vi "Limits Configurator.vi"() -> ()   [LabVIEW 2024]
doc: "Use this configurator to build a limits file based on specific sequence file. Uses the sequence file name to generate the limits file neame because they are paired."
uses:
  <vilib>/addons/_JKI Toolkits/State Machine/_JKI_lib_State_Machine.llb/Select State(s)_err__jki_lib_state_machine.vi
  <vilib>/addons/_JKI Toolkits/State Machine/_JKI_lib_State_Machine.llb/Periodic Trigger__ogtk__JKI-SM__jki_lib_state_machine.vi
  <userlib>/_OpenG.lib/file/file.llb/Convert File Extension (String)__ogtk.vi
  <userlib>/_OpenG.lib/file/file.llb/File Exists - Scalar__ogtk.vi
  <vilib>/Utility/file.llb/Write Delimited Spreadsheet (string).vi
  <vilib>/Utility/file.llb/Read Delimited Spreadsheet (string).vi
  <userlib>/_OpenG.lib/appcontrol/appcontrol.llb/openg_application_control.lvlib
  <userlib>/_OpenG.lib/file/file.llb/openg_file.lvlib
panel:
  in  "Remove Button":bool
  in  "Sequence File Path":path
  in  "Close Button":bool
  in  "Limits Table":i32(listbox)
  in  "Add Button":bool
  in  "Test Cases":u16(ring) items=["Connect Test", "PSU Test", "LED Test", "Firmware Test", "Shutdown"]
  # "LIMITS CONFIGURATOR"
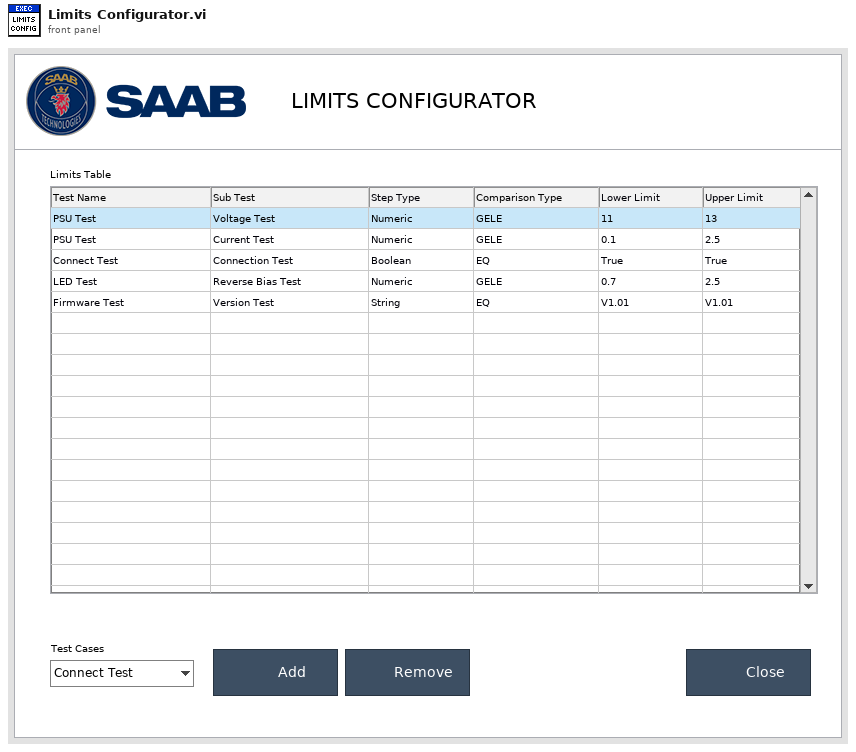
[diagram p1: front panel]
types:
  T1 = enum32{"Invalid", "Standard", "Closed", "Hidden", "Minimized", "Maximized"}
  T2 = enum32{"invalid app kind", "Development System", "Run Time System", "Student Edition", "Embedded LabVIEW", "Evaluation", "Custom"}
  T3 = enum8{"Enabled", "Disabled", "Disabled and Grayed Out"}
  T4 = cluster{"Core":cluster{"Current VI Reference":refnum<vi>, "Close Panel on Exit?":bool}, "Sequence File Path":path, "Limit Data Array":string[][], "Limits File Path":path}
  T5 = cluster{"Current VI Reference":refnum<vi>, "Close Panel on Exit?":bool}
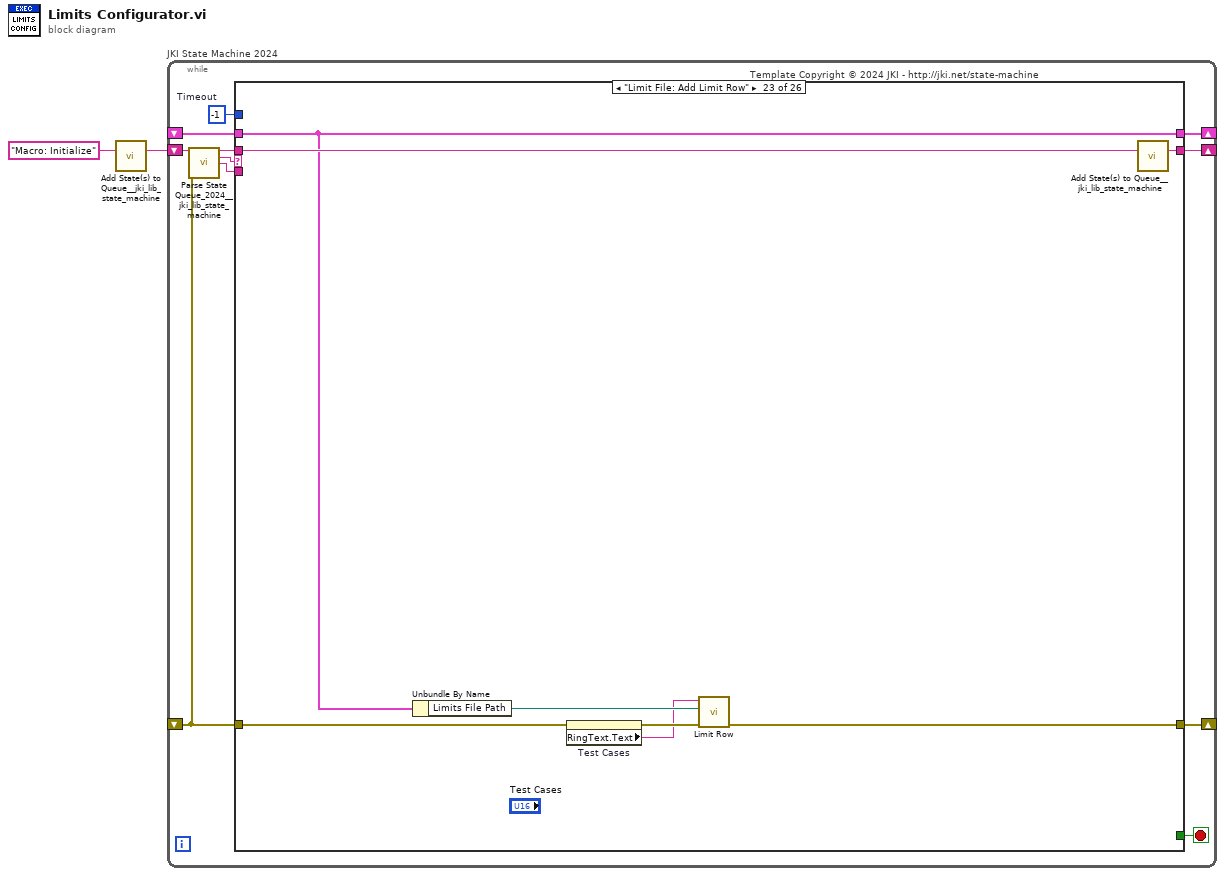
[diagram p0: block diagram]
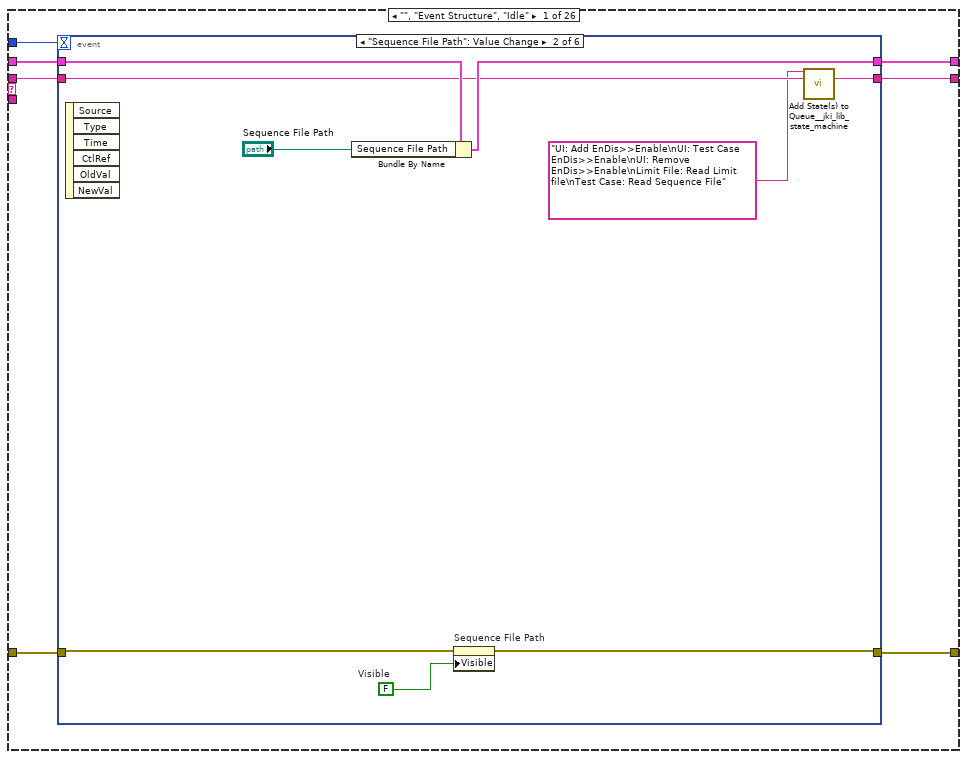
[diagram p2: hidden frame]
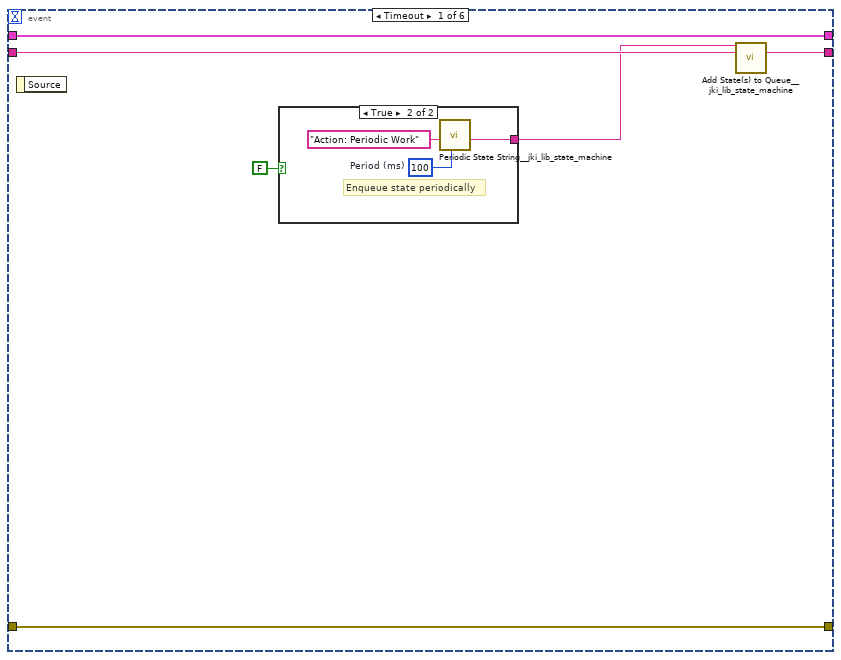
[diagram p3: hidden frame]
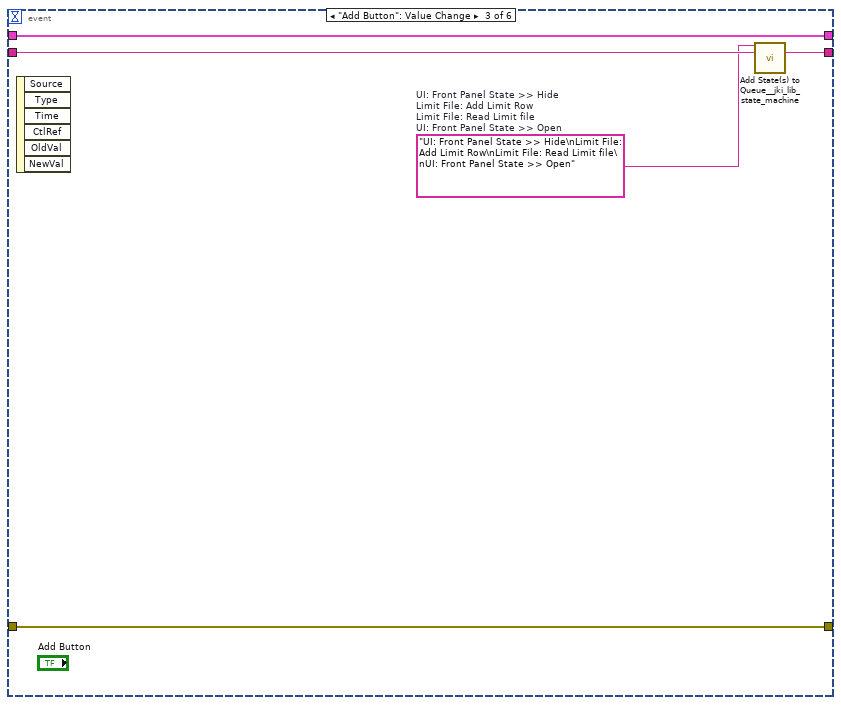
[diagram p5: hidden frame]
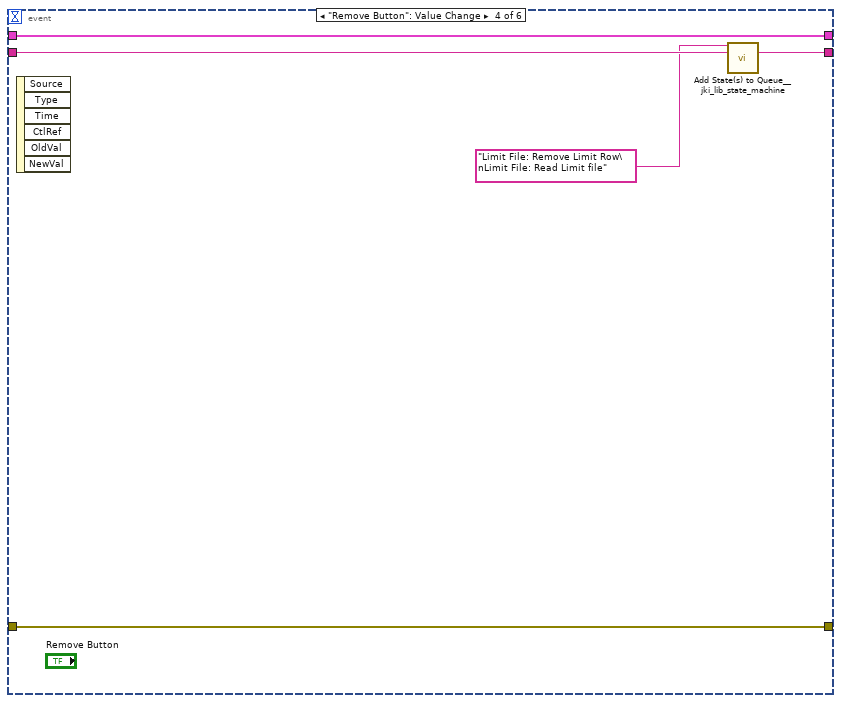
[diagram p6: hidden frame]
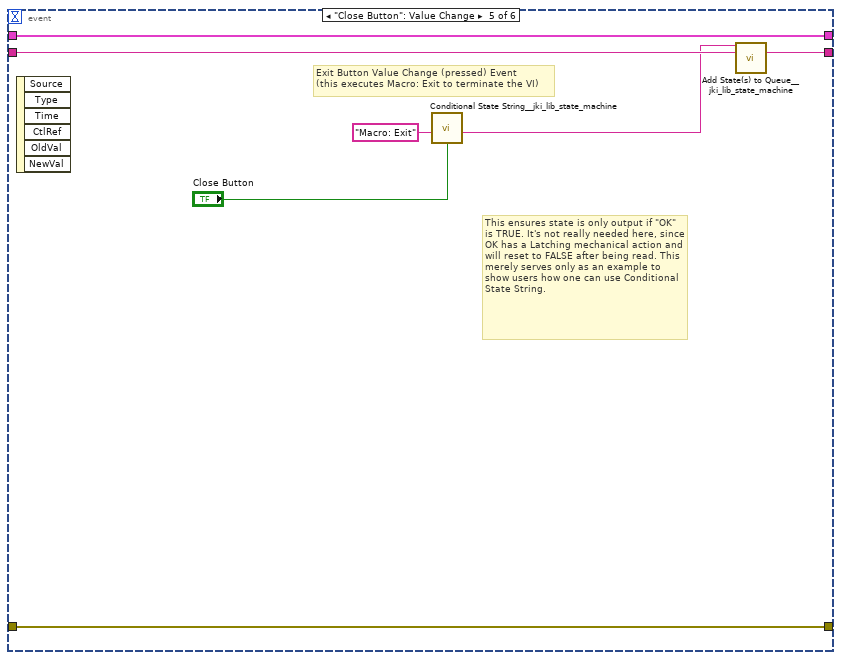
[diagram p7: hidden frame]
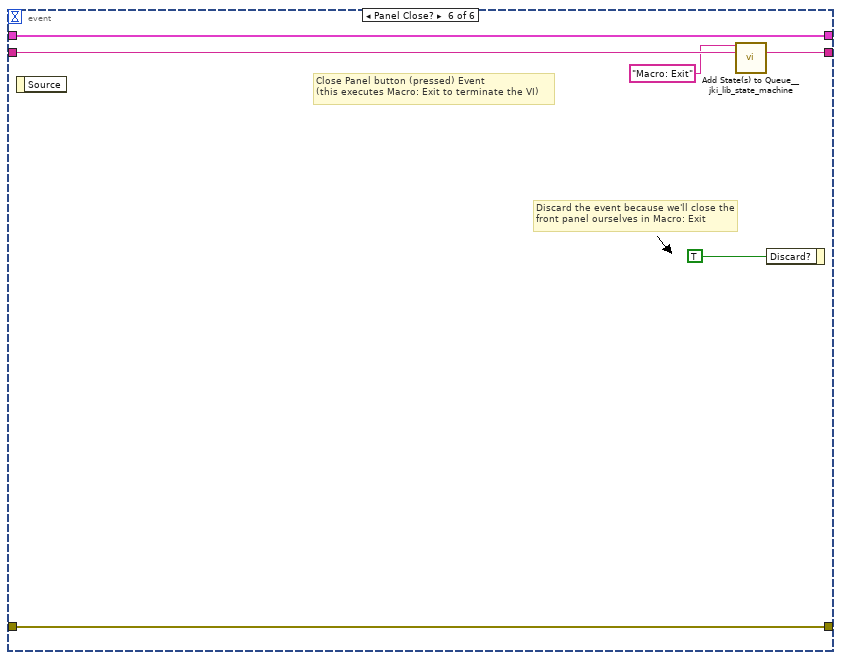
[diagram p8: hidden frame]
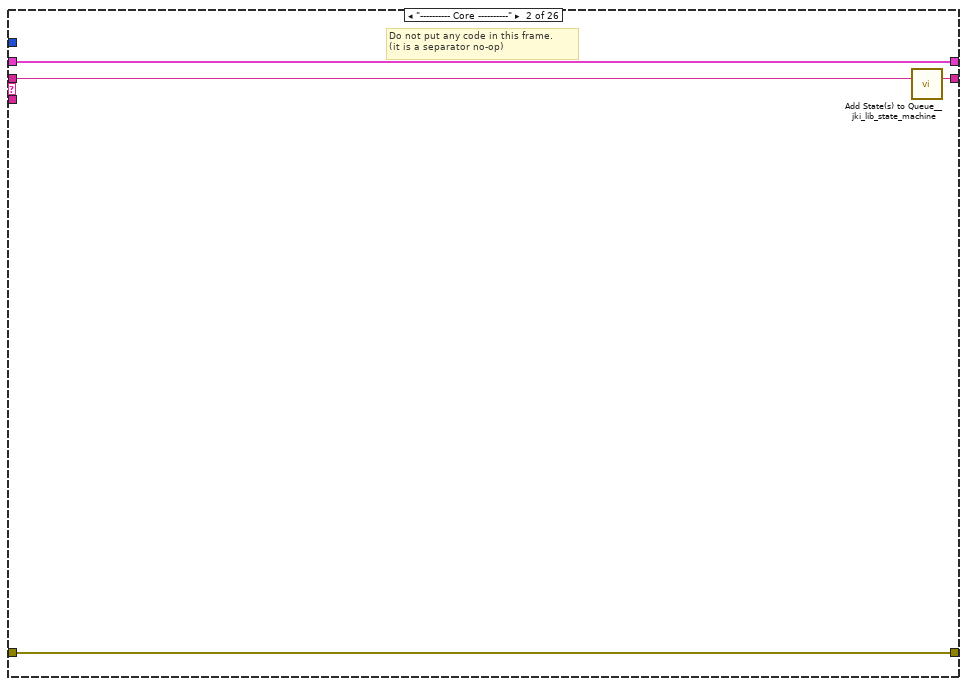
[diagram p9: hidden frame]
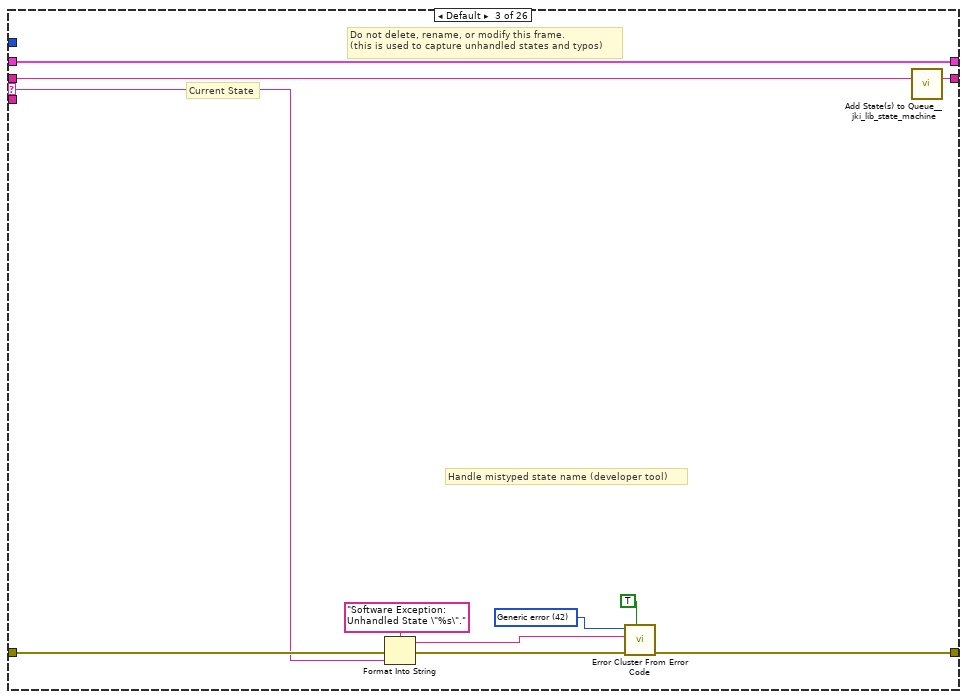
[diagram p10: hidden frame]
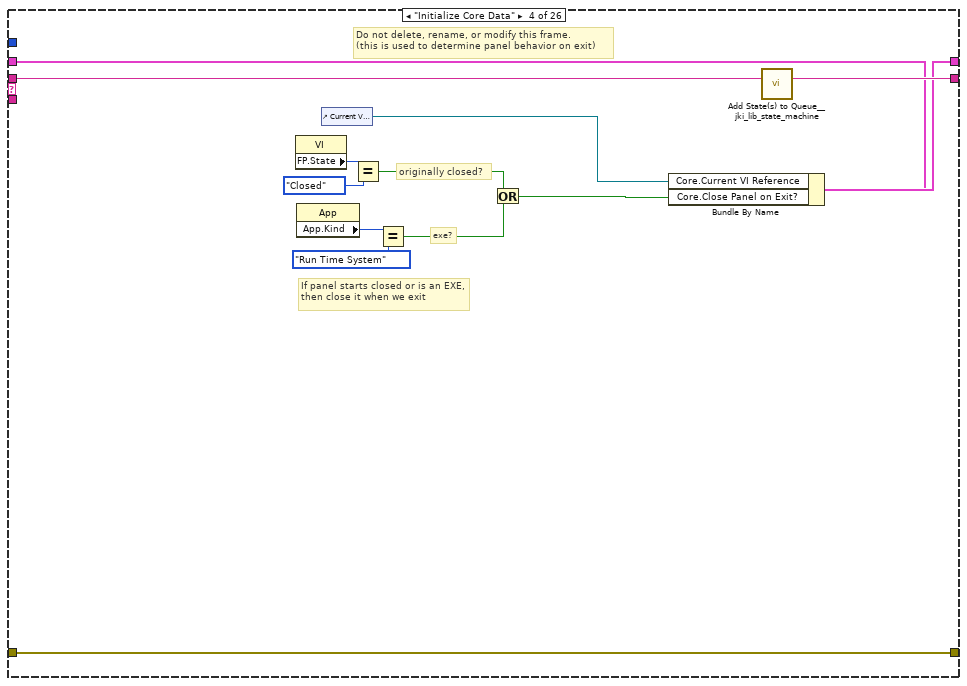
[diagram p11: hidden frame]
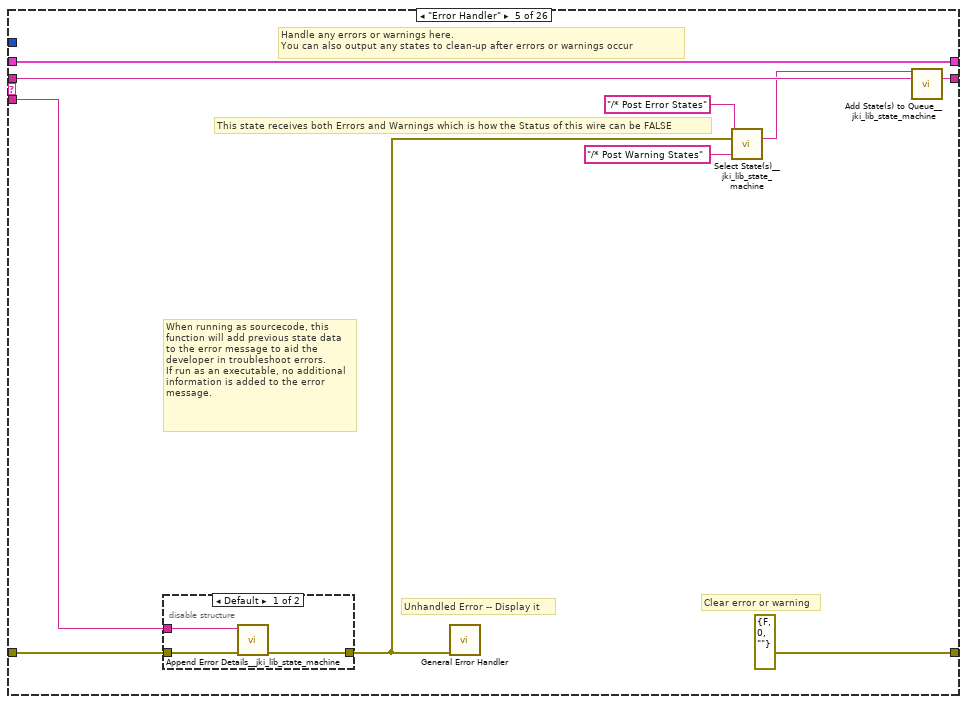
[diagram p12: hidden frame]
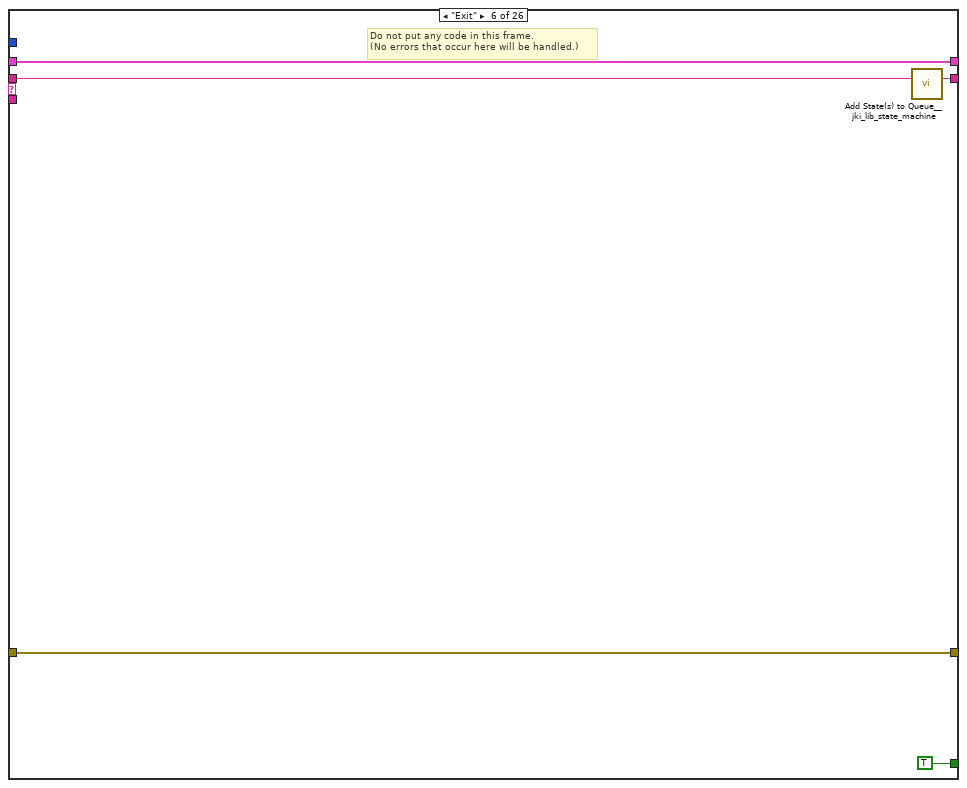
[diagram p14: hidden frame]
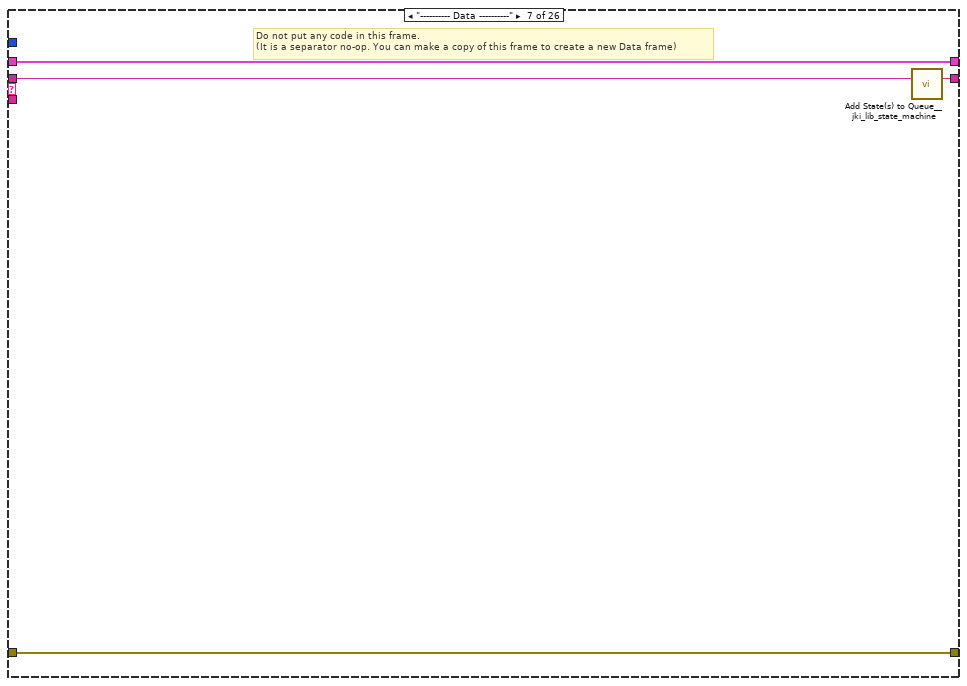
[diagram p15: hidden frame]
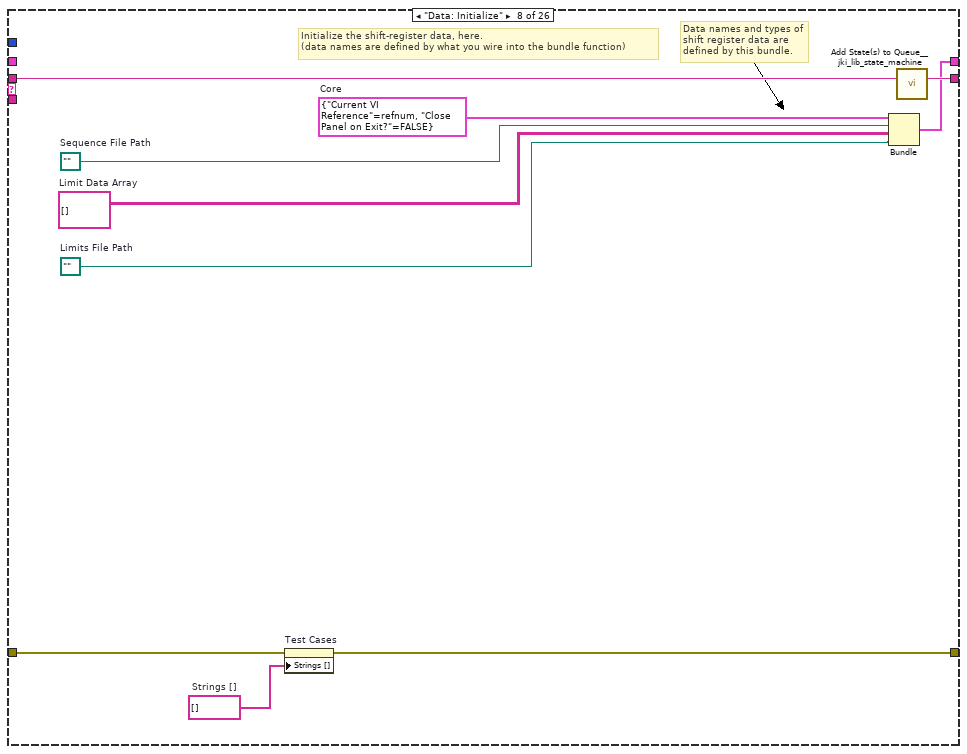
[diagram p16: hidden frame]
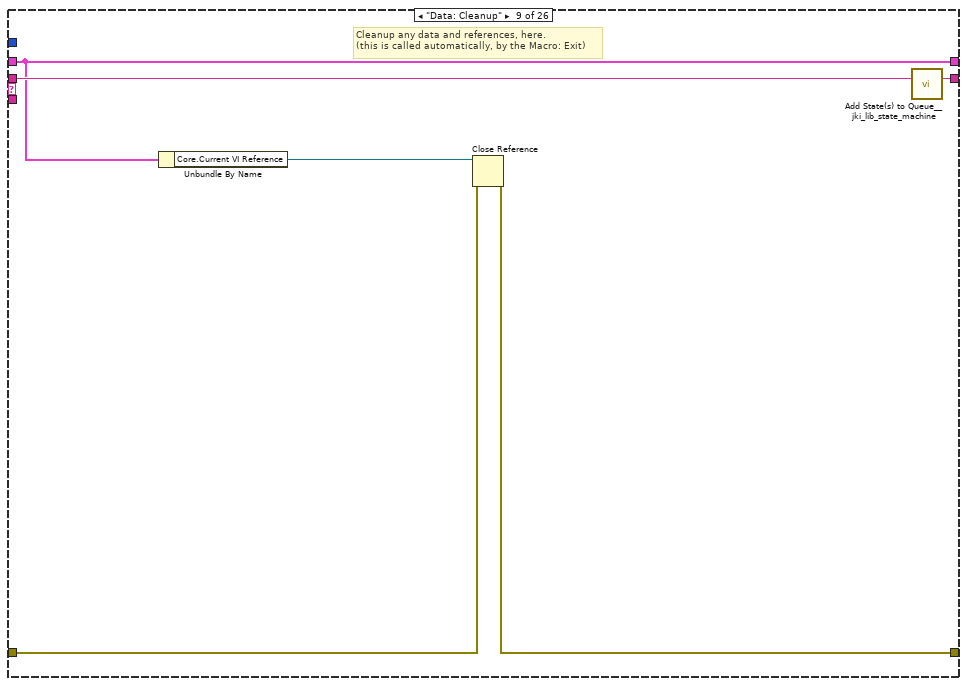
[diagram p17: hidden frame]
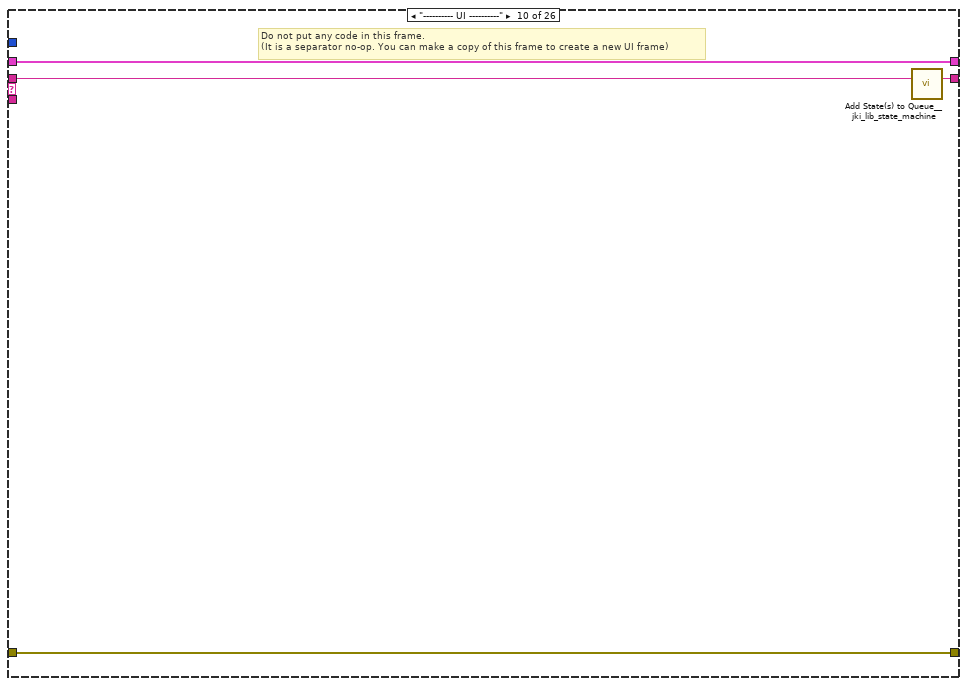
[diagram p18: hidden frame]
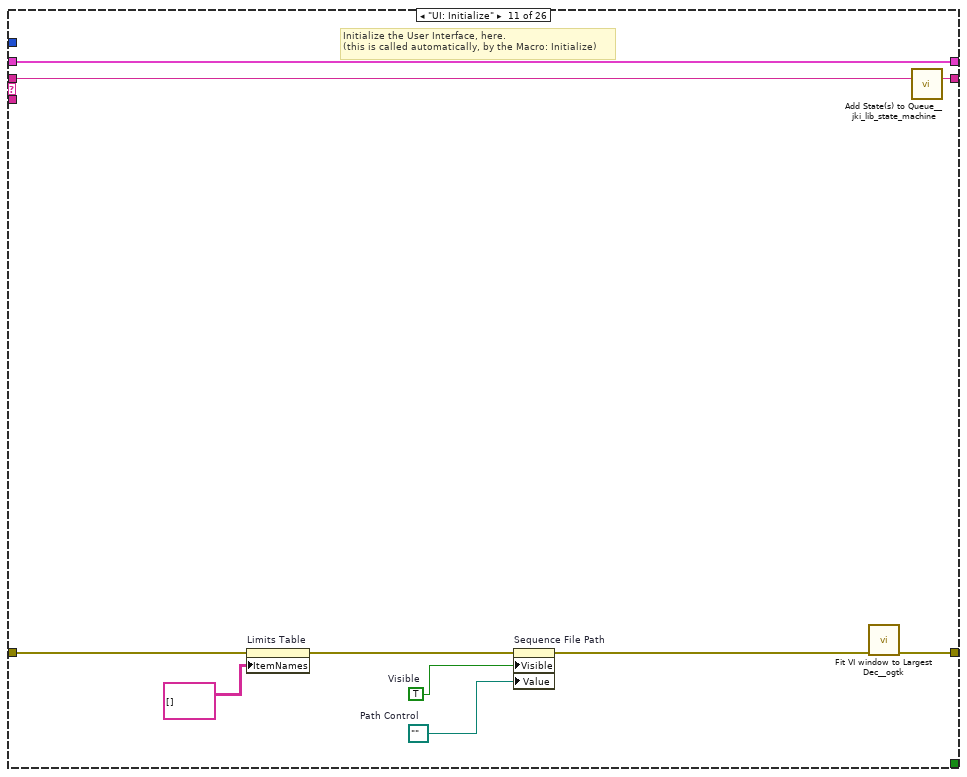
[diagram p19: hidden frame]
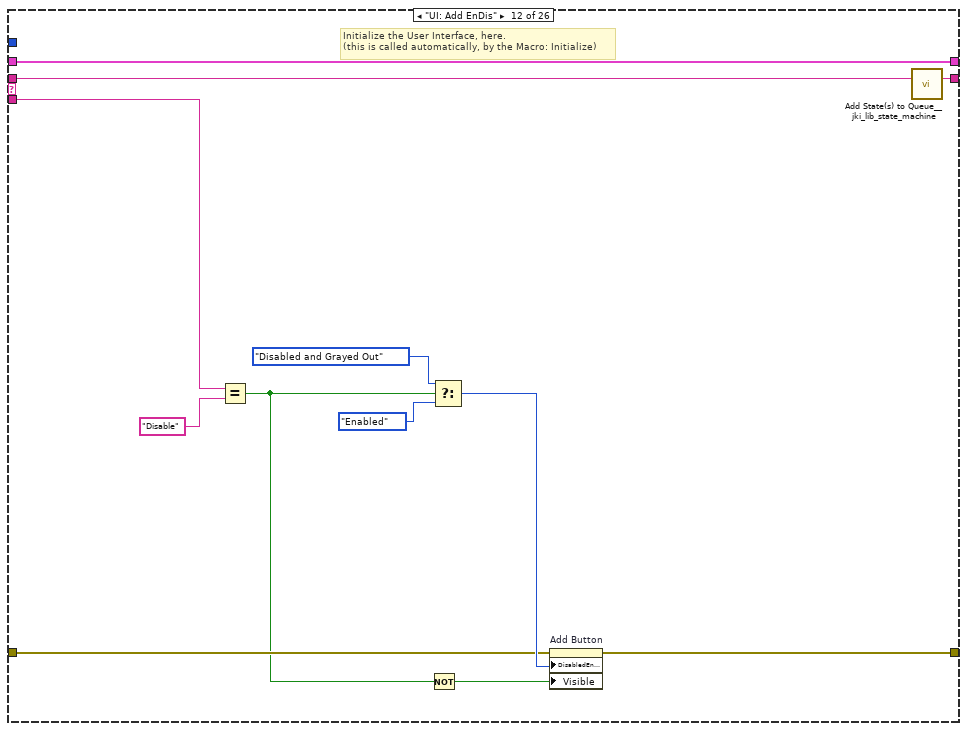
[diagram p20: hidden frame]
diagram:
  n1 = call <vilib>:"Add State(s) to Queue__jki_lib_state_machine.vi"("State(s) in (\"\")"="Macro: Initialize") -> ("States Out"=w2:string)  [unwired: 14 in]
  n2 = while "JKI State Machine 2024" {
    shift-right: [w6] -> _
    shift-left: _ -> [w5]
    shift-right: [w9] -> _
    shift-left: _ -> [w3]
    shift-right: [w8] -> _
    shift-left: w2 -> [w10]
    stop <- w7 stop-if-true
    w4 = -1  # Timeout
    # "Template Copyright © 2024 JKI - http://jki.net/state-machine"
    n3 = call <vilib>:"Parse State Queue_2024__jki_lib_state_machine.vi"("State Queue"=w10, "Error In (no error)"=w3) -> ("Remaining States"=w12:string, "Current State"=w13:string, "Arguments"=w11:string)  [unwired: 11 in]
    n4 = case shown="\"Limit File: Add Limit Row\"" w13 {
      selector: w13 -> [_ _ w66 _ _ _ _ _ _ _ _ _ _ _ _ _ _ _ _ _ _ _ _ _ _ _]
      tunnel: w12 -> [w20 w65 w70 w89 w99 w108 w112 w122 w128 w132 w142 w154 w166 w178 w182 w188 w199 w268 w273 w282 w286 w306 w328 w335 w351 w360]
      tunnel: w11 -> [_ _ _ _ w94 _ _ _ _ _ _ w146 w158 w170 _ w183 w193 _ _ _ _ _ _ _ _ _]
      tunnel: w5 -> [w18 w62 w68 w82 w96 w106 w109 _ w123 w129 w140 w152 w164 w176 w180 w186 w195 w265 w270 w280 w283 w289 w325 w333 w348 w353]
      tunnel: [w17 w63 w72 w86 errorcluster {"status"=FALSE, "code"=0, "source"=""} ("error out") w105 w110 w115 w124 w130 w139 w147 w159 w171 w179 w184 w196 w266 w271 w277 w284 w302 w326 w331 w349 w358] -> w9
      tunnel: w3 -> [w14 w63 w71 w86 w95 w105 w110 w114 w125 w130 w138 w145 w157 w169 w179 w185 w197 w266 w271 w277 w284 w304 w322 w332 w349 w357]
      tunnel: [w19 w64 w69 w88 w98 w107 w111 w121 w127 w131 w141 w153 w165 w177 w181 w187 w198 w267 w272 w281 w285 w305 w327 w334 w350 w359] -> w8
      tunnel: [_ _ _ _ _ TRUE _ _ _ _ _ _ _ _ _ _ _ _ _ _ _ _ _ _ _ _] -> w7
      tunnel: [w16 w62 w68 w87 w96 w106 w109 w120 w123 w129 w140 w152 w164 w176 w180 w186 w195 w265 w270 w280 w283 w288 w325 w333 w348 w353] -> w6
      tunnel: w4 -> [w15 _ _ _ _ _ _ _ _ _ _ _ _ _ _ _ _ _ _ _ _ _ _ _ _ _]
      frame "", "Event Structure", "Idle" {
        n5 = event shown="[1] \"Sequence File Path\": Value Change" {
          selector: _ -> [_ _ _ _ _ _]
          dyn-events: _ -> [_ _ _ _ _ _]
          timeout: w15 -> [_ _ _ _ _ _]
          tunnel: w20 -> [w26 w34 w41 w45 w55 w61]
          tunnel: [w25 w35 w42 w46 w54 w60] -> w19
          tunnel: w18 -> [w23 w38 w39 w47 w52 w58]
          tunnel: [w24 w32 w43 w48 w53 w59] -> w17
          tunnel: w14 -> [w24 w31 w43 w48 w53 w59]
          tunnel: [w23 w37 w39 w47 w52 w58] -> w16
          event Timeout {
            n6 = event-data() -> ()  [unwired: 1 in, 1 out]
            n7 = case shown="True" FALSE {
              tunnel: [_ w29] -> w22
              frame False {
              }
              frame True {
                w27 = u32 100  # Period (ms)
                # "Enqueue state periodically"
                n8 = call <vilib>:"Periodic State String__jki_lib_state_machine.vi"("Period (ms)"=w27, "State"="Action: Periodic Work") -> ("State Out"=w29:string)  [unwired: 9 in]
              }
            }
            n9 = call <vilib>:"Add State(s) to Queue__jki_lib_state_machine.vi"("State(s) in Front (\"\")"=w22, "State(s) in (\"\")"=w26) -> ("States Out"=w25:string)  [unwired: 13 in]
          }
          event "Sequence File Path": Value Change {
            w30 = FALSE  # Visible
            n10 = event-data() -> ()  [unwired: 1 in, 6 out]
            n11 = Bundle By Name(cluster=w38, "Sequence File Path"="Sequence File Path") -> (w37:T4)
            n12 = property on="Sequence File Path" class="Path"(error in=w31, "Visible"=w30) -> (error out=w32:errorcluster)  [unwired: 1 in, 1 out]
            n13 = call <vilib>:"Add State(s) to Queue__jki_lib_state_machine.vi"("State(s) in Front (\"\")"="UI: Add EnDis>>Enable\nUI: Test Case EnDis>>Enable\nUI: Remove EnDis>>Enable\nLimit File: Read Limit file\nTest Case: Read Sequence File", "State(s) in (\"\")"=w34) -> ("States Out"=w35:string)  [unwired: 13 in]
          }
          event "Add Button": Value Change {
            w40 = "UI: Front Panel State >> Hide\nLimit File: Add Limit Row\nLimit File: Read Limit file\nUI: Front Panel State >> Open"  # UI: Front Panel State >> Hide Limit File: Add Limit Row Limit File: Read Limit file UI: Front Panel State >> Open
            n14 = event-data() -> ()  [unwired: 1 in, 6 out]
            n15 = call <vilib>:"Add State(s) to Queue__jki_lib_state_machine.vi"("State(s) in Front (\"\")"=w40, "State(s) in (\"\")"=w41) -> ("States Out"=w42:string)  [unwired: 13 in]
          }
          event "Remove Button": Value Change {
            n16 = event-data() -> ()  [unwired: 1 in, 6 out]
            n17 = call <vilib>:"Add State(s) to Queue__jki_lib_state_machine.vi"("State(s) in Front (\"\")"="Limit File: Remove Limit Row\nLimit File: Read Limit file", "State(s) in (\"\")"=w45) -> ("States Out"=w46:string)  [unwired: 13 in]
          }
          event "Close Button": Value Change {
            # "This ensures state is only output if \"OK\" is TRUE. It's not really needed here, since OK has a Latching mechanical action and will reset to FALSE after being read. This merely serves only as an example to show users how one can use Conditional State String."
            # "Exit Button Value Change (pressed) Event\n(this executes Macro: Exit to terminate the VI)"
            n18 = event-data() -> ()  [unwired: 1 in, 6 out]
            n19 = call <vilib>:"Conditional State String__jki_lib_state_machine.vi"("Do State(s)?"="Close Button", "State"="Macro: Exit") -> ("State Out"=w50:string)  [unwired: 7 in]
            n20 = call <vilib>:"Add State(s) to Queue__jki_lib_state_machine.vi"("State(s) in Front (\"\")"=w50, "State(s) in (\"\")"=w55) -> ("States Out"=w54:string)  [unwired: 13 in]
          }
          event Panel Close? {
            # "Discard the event because we'll close the front panel ourselves in Macro: Exit"
            # "Close Panel button (pressed) Event\n(this executes Macro: Exit to terminate the VI)"
            n21 = event-data() -> ()  [unwired: 1 in, 1 out]
            n22 = call <vilib>:"Add State(s) to Queue__jki_lib_state_machine.vi"("State(s) in Front (\"\")"="Macro: Exit", "State(s) in (\"\")"=w61) -> ("States Out"=w60:string)  [unwired: 13 in]
            n23 = event-data("Discard?"=TRUE) -> ()  [unwired: 1 in, 1 out]
          }
        }
      }
      frame "---------- Core ----------" {
        # "Do not put any code in this frame.\n(it is a separator no-op)"
        n24 = call <vilib>:"Add State(s) to Queue__jki_lib_state_machine.vi"("State(s) in (\"\")"=w65) -> ("States Out"=w64:string)  [unwired: 14 in]
      }
      frame Default {
        w75 = 42 items=["No error", "Argument error", "Memory is full", "Out of zone", "End of file", "File already open", "Generic file I/O error", "File not found", "File permission error", "Disk is full", "Duplicate path", "Too many files open", "System feature not enabled", "Resource file not found", "Cannot add resource", "Resource not found", "Image not found", "Image memory error", "Pen does not exist", "Config type invalid", "Config token not found", "Config parse error", "Config memory error", "Bad external code format", "Bad external code offset", "External code not present", "Null window", "Destroy window error", "Null menu", "Print aborted", "Bad print record", "Print driver error", "Windows error during printing", "Memory error during printing", "Print dialog error", "Generic print error", "Invalid device refnum", "Device not found", "Device parameter error", "Device unit error", "Cannot open device", "Device call aborted", "Generic error", "Cancelled by user", "Object ID too low", "Object ID too high", "Object not in heap", "Unknown heap", "Unknown object (invalid DefProc)", "Unknown object (DefProc not in table)", "Message out of range", "Invalid (null) method", "Unknown message", "Manager call not supported", "Bad address", "Network operation in progress", "Network operation timed out", "Connection is busy", "Network attribute not supported", "Network error", "Address in use", "System out of memory", "Connection aborted", "Connection refused", "Not connected", "Already connected", "Connection closed", "Initialization error (interapplication manager)", "Bad occurrence", "Wait on unbound occurrence handler", "Occurrence queue overflow", "Datalog type conflict", "Unused", "Unrecognized type (interapplication manager)", "Memory corrupt", "Failed to make temporary DLL", "Old CIN version", "Drag socket not found", "Failed to load drop-object", "Failed to register OLE object", "Failed to release OLE object", "Format specifier type mismatch", "Unknown format specifier", "Too few format specifiers", "Too many format specifiers", "Scan failed", "Newer CIN version", "Error converting to variant", "Runtime menu error", "Password tampered", "Variant attribute not found", "Incompatible variant data type", "Event data is not available", "Event Store is not present", "Occurrence is not found", "Event Queue is not created", "Event info is not available", "Refnum passed is NULL", "Error retrieving Class GUID", "Error retrieving CoClass GUID", "Error retrieving TypeLib GUID.", "Bad built application magic bytes.", "Specific driver is different from the specific driver associated with the Logical Name.", "There is no session opened to the class driver.", "Max Error", "MAX - Error with config objects", "MAX - Error loading configuration", "MAX - Group not supported"]
        # "Current State"
        # "Do not delete, rename, or modify this frame.\n(this is used to capture unhandled states and typos)"
        # "Handle mistyped state name (developer tool)"
        n25 = Format Into String(format string="Software Exception: Unhandled State \"%s\"." ("message"), error in=w71, w66) -> (resulting string=w74:string, error out=w73:errorcluster)  [unwired: 1 in]
        n26 = call <vilib>:"Error Cluster From Error Code.vi"("show call chain? (False)"=TRUE, "error in (no error)"=w73, "error message (\"\")"=w74, "error code (0)"=w75) -> ("error out"=w72:errorcluster)  [unwired: 5 in]
        n27 = call <vilib>:"Add State(s) to Queue__jki_lib_state_machine.vi"("State(s) in (\"\")"=w70) -> ("States Out"=w69:string)  [unwired: 14 in]
      }
      frame "Initialize Core Data" {
        # "Do not delete, rename, or modify this frame.\n(this is used to determine panel behavior on exit)"
        # "originally closed?"
        # "exe?"
        # "If panel starts closed or is an EXE, then close it when we exit"
        n28 = property class="VI"() -> ("FP.State"=w79:T1)  [unwired: 2 in, 2 out]
        n29 = property class="App"() -> ("App.Kind"=w85:T2)  [unwired: 2 in, 2 out]
        n30 = control-ref of="Current VI Reference"() -> (w80:refnum<vi>)
        n31 = Equal?(x=w79, y=T1."Closed" ("Front Panel Window:State")) -> (x = y?=w77:bool)
        n32 = Equal?(x=w85, y=T2."Run Time System" ("Application:Kind")) -> (x = y?=w83:bool)
        n33 = Or(x=w77, y=w83) -> (x .or. y?=w81:bool)
        n34 = Bundle By Name(cluster=w82, "Core.Current VI Reference"=w80, "Core.Close Panel on Exit?"=w81) -> (w87:T4)
        n35 = call <vilib>:"Add State(s) to Queue__jki_lib_state_machine.vi"("State(s) in (\"\")"=w89) -> ("States Out"=w88:string)  [unwired: 14 in]
      }
      frame "Error Handler" {
        # "When running as sourcecode, this function will add previous state data to the error message to aid the developer in troubleshoot errors.\nIf run as an executable, no additional information is added to the error message."
        # "This state receives both Errors and Warnings which is how the Status of this wire can be FALSE"
        # "Unhandled Error -- Display it"
        # "Handle any errors or warnings here.\nYou can also output any states to clean-up after errors or warnings occur"
        # "Clear error or warning"
        n36 = disable-structure shown="Default" {
          disable-tunnel: w95 -> [w102 w103]
          disable-tunnel: w94 -> [w101 _]
          disable-tunnel: [w100 w103] -> w93
          frame condition #0 (active) {
            n37 = call <vilib>:"Append Error Details__jki_lib_state_machine.vi"("error in (no error)"=w102, "Previous State and Argument(s)"=w101) -> ("error out"=w100:errorcluster)  [unwired: 9 in]
          }
          frame condition #1 {
          }
        }
        n38 = call <vilib>:"General Error Handler.vi"("error in (no error)"=w93) -> ()  [unwired: 10 in, 5 out]
        n39 = call-poly <vilib>:"Select State(s)__jki_lib_state_machine.vi"("State(s) if True (\"\")"="/* Post Error States", "Select"=w93, "State(s) if False (\"\")"="/* Post Warning States") -> ("States Out"=w91:string)  [unwired: 12 in]
        n40 = call <vilib>:"Add State(s) to Queue__jki_lib_state_machine.vi"("State(s) in Front (\"\")"=w91, "State(s) in (\"\")"=w99) -> ("States Out"=w98:string)  [unwired: 13 in]
      }
      frame "Exit" {
        # "Do not put any code in this frame.\n(No errors that occur here will be handled.)"
        n41 = call <vilib>:"Add State(s) to Queue__jki_lib_state_machine.vi"("State(s) in (\"\")"=w108) -> ("States Out"=w107:string)  [unwired: 14 in]
      }
      frame "---------- Data ----------" {
        # "Do not put any code in this frame.\n(It is a separator no-op. You can make a copy of this frame to create a new Data frame)"
        n42 = call <vilib>:"Add State(s) to Queue__jki_lib_state_machine.vi"("State(s) in (\"\")"=w112) -> ("States Out"=w111:string)  [unwired: 14 in]
      }
      frame "Data: Initialize" {
        w113 = string[] []  # Strings []
        w116 = path ""  # Limits File Path
        w117 = string[][] []  # Limit Data Array
        w118 = path ""  # Sequence File Path
        w119 = T5 {"Current VI Reference"=refnum, "Close Panel on Exit?"=FALSE}  # Core
        # "Data names and types of shift register data are defined by this bundle."
        # "Initialize the shift-register data, here.\n(data names are defined by what you wire into the bundle function)"
        n43 = property on="Test Cases" class="Ring (strict)"(error in=w114, "Strings []"=w113) -> (error out=w115:errorcluster)  [unwired: 1 in, 1 out]
        n44 = Bundle("Core"=w119, "Sequence File Path"=w118, "Limit Data Array"=w117, "Limits File Path"=w116) -> (w120:T4)  [unwired: 1 in]
        n45 = call <vilib>:"Add State(s) to Queue__jki_lib_state_machine.vi"("State(s) in (\"\")"=w122) -> ("States Out"=w121:string)  [unwired: 14 in]
      }
      frame "Data: Cleanup" {
        # "Cleanup any data and references, here.\n(this is called automatically, by the Macro: Exit)"
        n46 = Unbundle By Name(w123) -> ("Core.Current VI Reference"=w126:refnum<vi>)
        n47 = Close Reference(reference=w126, error in (no error)=w125) -> (error out=w124:errorcluster)
        n48 = call <vilib>:"Add State(s) to Queue__jki_lib_state_machine.vi"("State(s) in (\"\")"=w128) -> ("States Out"=w127:string)  [unwired: 14 in]
      }
      frame "---------- UI ----------" {
        # "Do not put any code in this frame.\n(It is a separator no-op. You can make a copy of this frame to create a new UI frame)"
        n49 = call <vilib>:"Add State(s) to Queue__jki_lib_state_machine.vi"("State(s) in (\"\")"=w132) -> ("States Out"=w131:string)  [unwired: 14 in]
      }
      frame "UI: Initialize" {
        w133 = path ""  # Path Control
        w135 = TRUE  # Visible
        # "Initialize the User Interface, here.\n(this is called automatically, by the Macro: Initialize)"
        n50 = property on="Limits Table" class="MCListbox (strict)"(error in=w138, "ItemNames"=string[][] []) -> (error out=w136:errorcluster)  [unwired: 1 in, 1 out]
        n51 = property on="Sequence File Path" class="Path"(error in=w136, "Visible"=w135, "Value"=w133) -> (error out=w134:errorcluster)  [unwired: 1 in, 1 out]
        n52 = call <userlib>:"Fit VI window to Largest Dec__ogtk.vi"("error in (no error)"=w134) -> ("error out"=w139:errorcluster)  [unwired: 5 in, 1 out]
        n53 = call <vilib>:"Add State(s) to Queue__jki_lib_state_machine.vi"("State(s) in (\"\")"=w142) -> ("States Out"=w141:string)  [unwired: 14 in]
      }
      frame "UI: Add EnDis" {
        # "Initialize the User Interface, here.\n(this is called automatically, by the Macro: Initialize)"
        n54 = Equal?(x=w146, y="Disable") -> (x = y?=w143:bool)
        n55 = Not(x=w143) -> (.not. x?=w144:bool)
        n56 = Select(t=T3."Disabled and Grayed Out" ("Disabled"), s=w143, f=T3."Enabled" ("Disabled")) -> (s? t:f=w148:T3)
        n57 = property on="Add Button" class="Bool"(error in=w145, "DisabledEnum"=w148, "Visible"=w144) -> (error out=w147:errorcluster)  [unwired: 1 in, 1 out]
        n58 = call <vilib>:"Add State(s) to Queue__jki_lib_state_machine.vi"("State(s) in (\"\")"=w154) -> ("States Out"=w153:string)  [unwired: 14 in]
      }
      frame "UI: Remove EnDis" {
        # "Initialize the User Interface, here.\n(this is called automatically, by the Macro: Initialize)"
        n59 = Equal?(x=w158, y="Disable") -> (x = y?=w156:bool)
        n60 = Not(x=w156) -> (.not. x?=w155:bool)
        n61 = Select(t=T3."Disabled and Grayed Out" ("Disabled"), s=w156, f=T3."Enabled" ("Disabled")) -> (s? t:f=w160:T3)
        n62 = property on="Remove Button" class="Bool"(error in=w157, "DisabledEnum"=w160, "Visible"=w155) -> (error out=w159:errorcluster)  [unwired: 1 in, 1 out]
        n63 = call <vilib>:"Add State(s) to Queue__jki_lib_state_machine.vi"("State(s) in (\"\")"=w166) -> ("States Out"=w165:string)  [unwired: 14 in]
      }
      frame "UI: Test Case EnDis" {
        # "Initialize the User Interface, here.\n(this is called automatically, by the Macro: Initialize)"
        n64 = Equal?(x=w170, y="Disable") -> (x = y?=w168:bool)
        n65 = Not(x=w168) -> (.not. x?=w167:bool)
        n66 = Select(t=T3."Disabled and Grayed Out" ("Disabled"), s=w168, f=T3."Enabled" ("Disabled")) -> (s? t:f=w172:T3)
        n67 = property on="Test Cases" class="Ring (strict)"(error in=w169, "DisabledEnum"=w172, "Visible"=w167) -> (error out=w171:errorcluster)  [unwired: 1 in, 1 out]
        n68 = call <vilib>:"Add State(s) to Queue__jki_lib_state_machine.vi"("State(s) in (\"\")"=w178) -> ("States Out"=w177:string)  [unwired: 14 in]
      }
      frame "UI: Uninitialize" {
        # "Cleanup the User Interface, here.\n(this is called automatically, by the Macro: Exit)"
        n69 = call <vilib>:"Add State(s) to Queue__jki_lib_state_machine.vi"("State(s) in (\"\")"=w182) -> ("States Out"=w181:string)  [unwired: 14 in]
      }
      frame "UI: Cursor Set" {
        # "Argument"
        # "Set and Unset Cursor Busy.\n(Usage: \"UI: Cursor Set >> Busy|Idle\")"
        n70 = case shown="\"Idle\", Default" w183 {
          tunnel: w185 -> [w190 w192]
          tunnel: [w189 w191] -> w184
          frame "Idle", Default {
            n71 = call <vilib>:"Unset Busy.vi"("error in (no error)"=w190) -> ("error out"=w189:errorcluster)  [unwired: 10 in]
          }
          frame "Busy" {
            n72 = call <vilib>:"Set Busy.vi"("error in (no error)"=w192) -> ("error out"=w191:errorcluster)  [unwired: 9 in, 1 out]
          }
        }
        n73 = call <vilib>:"Add State(s) to Queue__jki_lib_state_machine.vi"("State(s) in (\"\")"=w188) -> ("States Out"=w187:string)  [unwired: 14 in]
      }
      frame "UI: Front Panel State" {
        # "Argument"
        # "Set Front Panel Open or Closed\n(Usage: \"UI: Front Panel State >> Open|Close\")"
        n74 = Unbundle By Name(w195) -> ("Core.Current VI Reference"=w194:refnum<vi>)
        n75 = case shown="\"Hidden\", \"Hide\"" w193 {
          tunnel: w197 -> [w205 w220 w231 w244 w257]
          tunnel: [w207 w221 w233 w246 w259] -> w196
          tunnel: w194 -> [w206 w218 w232 w245 w258]
          frame "Open", "Standard", Default {
            w200 = T1."Standard" ("State")
            n76 = property class="VI"(reference=w206, error in=w205) -> (reference out=w203:refnum<vi>, error out=w204:errorcluster, "FP.State"=w202:T1)
            n77 = Not Equal?(x=w202, y=w200) -> (x != y?=w201:bool)
            n78 = case shown="True" w201 {
              tunnel: [w211 w213] -> w207
              tunnel: w204 -> [w210 w213]
              tunnel: w203 -> [w209 _]
              tunnel: w200 -> [w208 _]
              frame True {
                n79 = invoke class="VI" method="FP.Open"(reference=w209, error in=w210, "Activate"=TRUE, "State"=w208) -> (error out=w211:errorcluster)  [unwired: 1 in, 4 out]
              }
              frame False {
              }
            }
          }
          frame "Close", "Closed" {
            n80 = property class="VI"(reference=w218, error in=w220) -> (reference out=w217:refnum<vi>, error out=w219:errorcluster, "FP.State"=w215:T1)
            n81 = Not Equal?(x=w215, y=T1."Closed" ("Front Panel Window:State")) -> (x != y?=w214:bool)
            n82 = case shown="True" w214 {
              tunnel: [w222 w225] -> w221
              tunnel: w219 -> [w222 w224]
              tunnel: w217 -> [_ w223]
              frame False {
              }
              frame True {
                n83 = invoke class="VI" method="FP.Close"(reference=w223, error in=w224) -> (error out=w225:errorcluster)  [unwired: 1 in, 2 out]
              }
            }
          }
          frame "Hidden", "Hide" {
            w226 = T1."Hidden" ("State")
            n84 = property class="VI"(reference=w232, error in=w231) -> (reference out=w229:refnum<vi>, error out=w230:errorcluster, "FP.State"=w228:T1)
            n85 = Not Equal?(x=w228, y=w226) -> (x != y?=w227:bool)
            n86 = case shown="True" w227 {
              tunnel: [w237 w238] -> w233
              tunnel: w230 -> [w236 w238]
              tunnel: w229 -> [w235 _]
              tunnel: w226 -> [w234 _]
              frame True {
                n87 = invoke class="VI" method="FP.Open"(reference=w235, error in=w236, "State"=w234) -> (error out=w237:errorcluster)  [unwired: 2 in, 4 out]
              }
              frame False {
              }
            }
          }
          frame "Minimize", "Minimized" {
            w239 = T1."Minimized" ("State")
            n88 = property class="VI"(reference=w245, error in=w244) -> (reference out=w242:refnum<vi>, error out=w243:errorcluster, "FP.State"=w241:T1)
            n89 = Not Equal?(x=w241, y=w239) -> (x != y?=w240:bool)
            n90 = case shown="True" w240 {
              tunnel: [w250 w251] -> w246
              tunnel: w243 -> [w249 w251]
              tunnel: w242 -> [w248 _]
              tunnel: w239 -> [w247 _]
              frame True {
                n91 = invoke class="VI" method="FP.Open"(reference=w248, error in=w249, "State"=w247) -> (error out=w250:errorcluster)  [unwired: 2 in, 4 out]
              }
              frame False {
              }
            }
          }
          frame "Maximize", "Maximized" {
            w252 = T1."Maximized" ("State")
            n92 = property class="VI"(reference=w258, error in=w257) -> (reference out=w255:refnum<vi>, error out=w256:errorcluster, "FP.State"=w254:T1)
            n93 = Not Equal?(x=w254, y=w252) -> (x != y?=w253:bool)
            n94 = case shown="True" w253 {
              tunnel: [w263 w264] -> w259
              tunnel: w256 -> [w262 w264]
              tunnel: w255 -> [w261 _]
              tunnel: w252 -> [w260 _]
              frame True {
                n95 = invoke class="VI" method="FP.Open"(reference=w261, error in=w262, "State"=w260) -> (error out=w263:errorcluster)  [unwired: 2 in, 4 out]
              }
              frame False {
              }
            }
          }
        }
        n96 = call <vilib>:"Add State(s) to Queue__jki_lib_state_machine.vi"("State(s) in (\"\")"=w199) -> ("States Out"=w198:string)  [unwired: 14 in]
      }
      frame "---------- Macro ----------" {
        # "Do not put any code in this frame.\n(It is a separator no-op. You can make a copy of this frame to create a new Macro frame)"
        n97 = call <vilib>:"Add State(s) to Queue__jki_lib_state_machine.vi"("State(s) in (\"\")"=w268) -> ("States Out"=w267:string)  [unwired: 14 in]
      }
      frame "Macro: Initialize" {
        w269 = "Data: Initialize\nInitialize Core Data\nUI: Initialize\nUI: Front Panel State >> Open\nUI: Add EnDis>>Disable\nUI: Test Case EnDis>>Disable\nUI: Remove EnDis>>Disable"  # Data: Initialize Initialize Core Data UI: Initialize UI: Front Panel State >> Open UI: Add EnDis>>Disable UI: Test Case EnDis>>Disable UI: Remove EnDis>>Disable
        # "Initialization Macro\n(This is called once, when the VI starts)"
        n98 = call <vilib>:"Add State(s) to Queue__jki_lib_state_machine.vi"("State(s) in Front (\"\")"=w269, "State(s) in (\"\")"=w273) -> ("States Out"=w272:string)  [unwired: 13 in]
      }
      frame "Macro: Exit" {
        # "Exit Macro\n(This is called once, when the VI exits)"
        n99 = Unbundle By Name(w280) -> ("Core.Close Panel on Exit?"=w275:bool)
        n100 = call <vilib>:"Conditional State String__jki_lib_state_machine.vi"("Do State(s)?"=w275, "State"="UI: Front Panel State >> Close") -> ("State Out"=w274:string)  [unwired: 7 in]
        n101 = call <vilib>:"Add State(s) to Queue__jki_lib_state_machine.vi"("State(s) in (\"\")"=w274, "State(s) at Back (\"\")"="UI: Uninitialize\nData: Cleanup\nExit") -> ("States Out"=w278:string)  [unwired: 13 in]
        n102 = call <vilib>:"Add State(s) to Queue__jki_lib_state_machine.vi"("State(s) in Front (\"\")"=w278, "State(s) in (\"\")"=w282) -> ("States Out"=w281:string)  [unwired: 13 in]
      }
      frame "---------- Limit File ----------" {
        # "Template Separator\n(You can make a copy of, or modify, this frame)"
        n103 = call <vilib>:"Add State(s) to Queue__jki_lib_state_machine.vi"("State(s) in (\"\")"=w286) -> ("States Out"=w285:string)  [unwired: 14 in]
      }
      frame "Limit File: Read Limit file" {
        w300 = FALSE  # Key Focus
        # "Your code here.\n(You can make a copy of, or modify, this frame)"
        n104 = Unbundle By Name(w289) -> ("Sequence File Path"=w291:path)
        n105 = Strip Path(path=w291) -> (stripped path=w299:path, name=w298:string)
        n106 = call-poly <userlib>:"Convert File Extension__ogtk.vi"("file name"=w298) -> ("new filename"=w297:string)  [unwired: 1 in, 1 out]
        n107 = Concatenate Strings(w297, " Limits.csv") -> (w294:string)
        n108 = Strip Path(path=w299) -> (stripped path=w296:path)  [unwired: 1 out]
        n109 = Concatenate Strings("Limits\\", w294) -> (w295:string)
        n110 = Build Path(base path=w296, name or relative path=w295) -> (appended path=w287:path)
        n111 = call-poly <userlib>:"File Exists__ogtk.vi"("file path"=w287) -> ("exists"=w290:bool)  [unwired: 6 in, 1 out]
        n112 = case shown="False" w290 {
          tunnel: w304 -> [w310 w320]
          tunnel: [w311 w317] -> w303
          tunnel: [w312 w315] -> w301
          tunnel: w287 -> [w309 w313]
          frame False {
            w307 = ","  # delimiter (\t)
            w312 = string[][] []  # all rows
            # "Limits Fille"
            n113 = call-poly <vilib>:"Write Delimited Spreadsheet.vi"("file path (dialog if empty)"=w309, "1D data"=string[] ["Test Case", "Sub Test", "Step Type", "Comparison type", "Lower Limit", "Higher Limit"], "error in (no error)"=w310, "delimiter (\\t)"=w307) -> ("error out"=w311:errorcluster)  [unwired: 10 in, 1 out]
          }
          frame True {
            n114 = call-poly <vilib>:"Read Delimited Spreadsheet.vi"("file path (dialog if empty)"=w313, "start of read offset (chars.:0)"=0, "error in (no error)"=w320, "delimiter (\\t)"="," ("delimiter (\\t)")) -> ("all rows"=w316:string[][], "error out"=w317:errorcluster)  [unwired: 6 in, 4 out]
            n115 = Delete From Array(array=w316, index (row)=0) -> (array with subset deleted=w315:string[][])  [unwired: 2 in, 1 out]
          }
        }
        n116 = Bundle By Name(cluster=w289, "Limits File Path"=w287) -> (w288:T4)
        n117 = property on="Limits Table" class="MCListbox (strict)"(error in=w303, "ItemNames"=w301, "Key Focus"=w300) -> (error out=w302:errorcluster)  [unwired: 1 in, 1 out]
        n118 = call <vilib>:"Add State(s) to Queue__jki_lib_state_machine.vi"("State(s) in (\"\")"=w306) -> ("States Out"=w305:string)  [unwired: 14 in]
      }
      frame "Limit File: Add Limit Row" {
        n119 = Unbundle By Name(w325) -> ("Limits File Path"=w324:path)
        n120 = property on="Test Cases" class="Ring (strict)"(error in=w322) -> (error out=w323:errorcluster, "RingText.Text"=w321:string)  [unwired: 1 in, 1 out]
        n121 = call "Limit Row.vi"("error in (no error)"=w323, "Limit File Path"=w324, "Test Case"=w321) -> ("error out"=w326:errorcluster)  [unwired: 8 in]
        n122 = call <vilib>:"Add State(s) to Queue__jki_lib_state_machine.vi"("State(s) in (\"\")"=w328) -> ("States Out"=w327:string)  [unwired: 14 in]
      }
      frame "Limit File: Remove Limit Row" {
        w330 = "Warning this will delete the selected row\nAre you sure?"  # message
        n123 = Two Button Dialog(message=w330) -> (T button?=w329:bool)  [unwired: 2 in]
        n124 = case shown="True" w329 {
          tunnel: w333 -> [_ w347]
          tunnel: w332 -> [w336 w346]
          tunnel: [w336 w337] -> w331
          frame False {
          }
          frame True {
            w338 = ","  # delimiter (\t)
            n125 = Unbundle By Name(w347) -> ("Limits File Path"=w341:path)
            n126 = call-poly <vilib>:"Read Delimited Spreadsheet.vi"("file path (dialog if empty)"=w341, "error in (no error)"=w346, "delimiter (\\t)"=w338) -> ("all rows"=w344:string[][], "error out"=w345:errorcluster)  [unwired: 7 in, 4 out]
            n127 = property on="Limits Table" class="MCListbox (strict)"(error in=w345) -> (error out=w339:errorcluster, "FocusRow"=w343:i32)  [unwired: 1 in, 1 out]
            n128 = Increment(x=w343) -> (x+1=w342:i32)
            n129 = Delete From Array(array=w344, index (row)=w342) -> (array with subset deleted=w340:string[][])  [unwired: 2 in, 1 out]
            n130 = call-poly <vilib>:"Write Delimited Spreadsheet.vi"("file path (dialog if empty)"=w341, "2D data"=w340, "error in (no error)"=w339, "delimiter (\\t)"=w338) -> ("error out"=w337:errorcluster)  [unwired: 10 in, 1 out]
          }
        }
        n131 = call <vilib>:"Add State(s) to Queue__jki_lib_state_machine.vi"("State(s) in (\"\")"=w335) -> ("States Out"=w334:string)  [unwired: 14 in]
      }
      frame "---------- Test Case ----------" {
        # "Template Separator\n(You can make a copy of, or modify, this frame)"
        n132 = call <vilib>:"Add State(s) to Queue__jki_lib_state_machine.vi"("State(s) in (\"\")"=w351) -> ("States Out"=w350:string)  [unwired: 14 in]
      }
      frame "Test Case: Read Sequence File" {
        w354 = ","  # delimiter (\t)
        # "Template Separator\n(You can make a copy of, or modify, this frame)"
        n133 = Unbundle By Name(w353) -> ("Sequence File Path"=w352:path)
        n134 = call-poly <vilib>:"Read Delimited Spreadsheet.vi"("file path (dialog if empty)"=w352, "error in (no error)"=w357, "delimiter (\\t)"=w354) -> ("first row"=w356:string[], "error out"=w355:errorcluster)  [unwired: 7 in, 4 out]
        n135 = property on="Test Cases" class="Ring (strict)"(error in=w355, "Strings []"=w356) -> (error out=w358:errorcluster)  [unwired: 1 in, 1 out]
        n136 = call <vilib>:"Add State(s) to Queue__jki_lib_state_machine.vi"("State(s) in (\"\")"=w360) -> ("States Out"=w359:string)  [unwired: 14 in]
      }
    }
  }
